vi "Word_Get_Table_Range.vi"(4 "end column":i32, 5 "start column":i32, 6 "end row":i32, 7 "start row":i32, 8 "error in":errorcluster, 9 "borders and shading":T1={"outside line style"=1, "outside color"=4278190080, "outside line width"=2, "inside line style"=1, "inside color"=4278190080, "inside line width"=2, "background pattern color"=4278190080} {"inside line style" items=["wdLineStyleNone", "wdLineStyleSingle", "wdLineStyleDot", "wdLineStyleDashSmallGap", "wdLineStyleDashLargeGap", "wdLineStyleDashDot", "wdLineStyleDashDotDot", "wdLineStyleDouble", "wdLineStyleTriple", "wdLineStyleThinThickSmallGap", "wdLineStyleThickThinSmallGap", "wdLineStyleThinThickThinSmallGap", "wdLineStyleThinThickMedGap", "wdLineStyleThickThinMedGap", "wdLineStyleThinThickThinMedGap", "wdLineStyleThinThickLargeGap", "wdLineStyleThickThinLargeGap", "wdLineStyleThinThickThinLargeGap", "wdLineStyleSingleWavy", "wdLineStyleDoubleWavy", "wdLineStyleDashDotStroked", "wdLineStyleEmboss3D", "wdLineStyleEngrave3D", "wdLineStyleOutset", "wdLineStyleInset"]; "inside line width" items=["wdLineWidth025pt"=2, "wdLineWidth050pt"=4, "wdLineWidth075pt"=6, "wdLineWidth100pt"=8, "wdLineWidth150pt"=12, "wdLineWidth225pt"=18, "wdLineWidth300pt"=24, "wdLineWidth450pt"=36, "wdLineWidth600pt"=48]; "outside line width" items=["wdLineWidth025pt"=2, "wdLineWidth050pt"=4, "wdLineWidth075pt"=6, "wdLineWidth100pt"=8, "wdLineWidth150pt"=12, "wdLineWidth225pt"=18, "wdLineWidth300pt"=24, "wdLineWidth450pt"=36, "wdLineWidth600pt"=48]; "outside line style" items=["wdLineStyleNone", "wdLineStyleSingle", "wdLineStyleDot", "wdLineStyleDashSmallGap", "wdLineStyleDashLargeGap", "wdLineStyleDashDot", "wdLineStyleDashDotDot", "wdLineStyleDouble", "wdLineStyleTriple", "wdLineStyleThinThickSmallGap", "wdLineStyleThickThinSmallGap", "wdLineStyleThinThickThinSmallGap", "wdLineStyleThinThickMedGap", "wdLineStyleThickThinMedGap", "wdLineStyleThinThickThinMedGap", "wdLineStyleThinThickLargeGap", "wdLineStyleThickThinLargeGap", "wdLineStyleThinThickThinLargeGap", "wdLineStyleSingleWavy", "wdLineStyleDoubleWavy", "wdLineStyleDashDotStroked", "wdLineStyleEmboss3D", "wdLineStyleEngrave3D", "wdLineStyleOutset", "wdLineStyleInset"]}, 10 "table":refnum<k7>, 11 "Word._Application":refnum<k7>) -> (0 "error out":errorcluster)   [LabVIEW 2010, in "NI_ReportGenerationToolkit.lvlib"]
uses:
  <vilib>/addons/_office/NI_ReportGenerationToolkit.lvlib
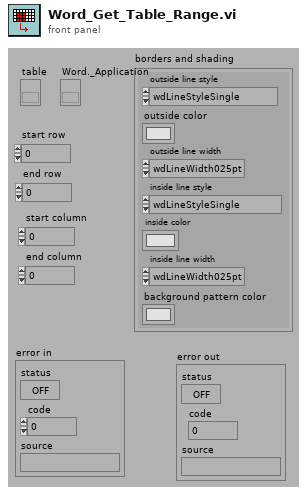
[diagram p1: front panel]
types:
  T1 = cluster{"outside line style":i32, "outside color":u32, "outside line width":i32, "inside line style":i32, "inside color":u32, "inside line width":i32, "background pattern color":u32}
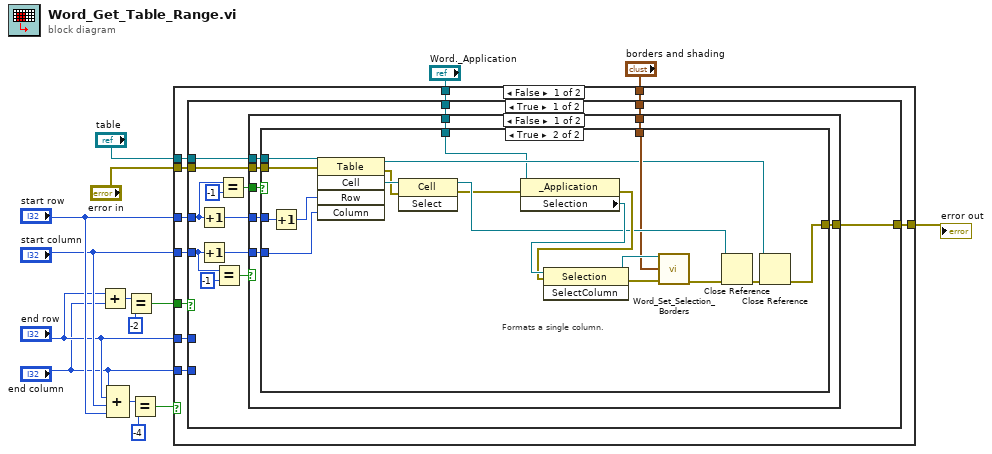
[diagram p0: block diagram]
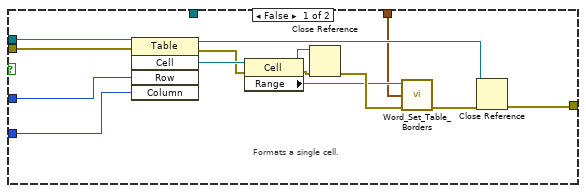
[diagram p2: hidden frame]
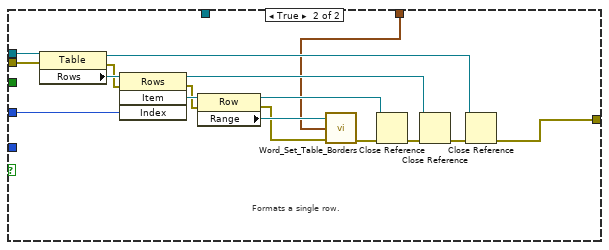
[diagram p3: hidden frame]
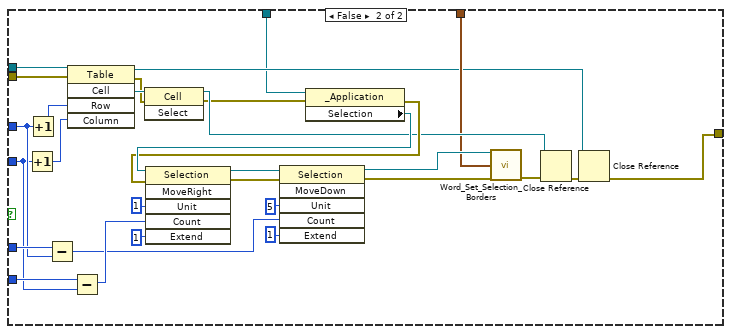
[diagram p4: hidden frame]
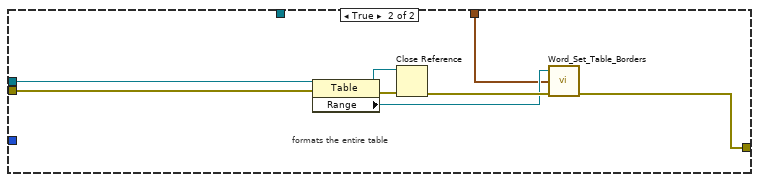
[diagram p5: hidden frame]
diagram:
  n1 = Add(x="end row", y="end column") -> (x+y=w13:i32)
  n2 = Compound Arithmetic op=ADD("end column", "end row", "start column", "start row") -> (w15:i32)
  n3 = Equal?(x=w13, y=-2) -> (x = y?=w4:bool)
  n4 = Equal?(x=w15, y=-4) -> (x = y?=w3:bool)
  n5 = case shown="False" w3 {
    tunnel: "start column" -> [w25 _]
    tunnel: "start row" -> [w24 _]
    tunnel: "end row" -> [w23 _]
    tunnel: "end column" -> [w22 _]
    tunnel: [w21 w128] -> w5
    tunnel: "table" -> [w20 w134]
    tunnel: "error in" -> [w19 w133]
    tunnel: "borders and shading" -> [w18 w127]
    tunnel: w4 -> [w17 _]
    tunnel: "Word._Application" -> [w16 _]
    frame False {
      n6 = case shown="True" w17 {
        tunnel: w25 -> [w32 w109]
        tunnel: w24 -> [w29 w110]
        tunnel: w23 -> [_ w112]
        tunnel: w22 -> [_ w111]
        tunnel: [w38 w104] -> w21
        tunnel: w20 -> [w37 w126]
        tunnel: w19 -> [w34 w125]
        tunnel: w18 -> [w27 w100]
        tunnel: w16 -> [w26 w97]
        frame True {
          n7 = Increment(x=w29) -> (x+1=w36:i32)
          n8 = Increment(x=w32) -> (x+1=w35:i32)
          n9 = Equal?(x=w32, y=-1) -> (x = y?=w33:bool)
          n10 = Equal?(x=w29, y=-1) -> (x = y?=w28:bool)
          n11 = case shown="False" w33 {
            tunnel: [w46 w85] -> w38
            tunnel: w37 -> [w45 w96]
            tunnel: w36 -> [w44 w94]
            tunnel: w35 -> [w43 _]
            tunnel: w34 -> [w42 w90]
            tunnel: w28 -> [w41 _]
            tunnel: w27 -> [w40 w80]
            tunnel: w26 -> [w39 _]
            frame False {
              n12 = case shown="True" w41 {
                tunnel: [w52 w72] -> w46
                tunnel: w45 -> [w58 w79]
                tunnel: w44 -> [w57 w77]
                tunnel: w43 -> [w56 w76]
                tunnel: w42 -> [w54 w78]
                tunnel: w40 -> [w47 w65]
                tunnel: w39 -> [_ w62]
                frame False {
                  # "Formats a single cell."
                  n13 = invoke class="Table" method="Cell"(reference=w58, error in=w54, "Row"=w57, "Column"=w56) -> (reference out=w51:refnum<k7>, error out=w53:errorcluster, "Cell"=w55:refnum<k7>)  [unwired: 1 in, 2 out]
                  n14 = property class="Cell"(reference=w55, error in=w53) -> (reference out=w60:refnum<k7>, error out=w59:errorcluster, "Range"=w48:refnum<k7>)
                  n15 = Close Reference(reference=w60, error in (no error)=w59) -> (error out=w49:errorcluster)
                  n16 = call <vilib>:"Word_Set_Table_Borders.vi"("range"=w48, "borders and shading"=w47, "error in"=w49) -> ("error out"=w50:errorcluster)  [unwired: 12 out]
                  n17 = Close Reference(reference=w51, error in (no error)=w50) -> (error out=w52:errorcluster)
                }
                frame True {
                  # "Formats a single column."
                  n18 = Increment(x=w77) -> (x+1=w61:i32)
                  n19 = invoke class="Table" method="Cell"(reference=w79, error in=w78, "Row"=w61, "Column"=w76) -> (reference out=w64:refnum<k7>, error out=w74:errorcluster, "Cell"=w75:refnum<k7>)  [unwired: 1 in, 2 out]
                  n20 = invoke class="Cell" method="Select"(reference=w75, error in=w74) -> (reference out=w69:refnum<k7>, error out=w63:errorcluster)  [unwired: 1 in, 1 out]
                  n21 = property class="_Application"(reference=w62, error in=w63) -> (error out=w70:errorcluster, "Selection"=w71:refnum<k7>)  [unwired: 1 out]
                  n22 = invoke class="Selection" method="SelectColumn"(reference=w71, error in=w70) -> (reference out=w66:refnum<k7>, error out=w68:errorcluster)  [unwired: 1 in, 1 out]
                  n23 = call <vilib>:"Word_Set_Selection_Borders.vi"("Word.Selection"=w66, "borders and shading"=w65, "error in"=w68) -> ("error out"=w67:errorcluster)  [unwired: 12 out]
                  n24 = Close Reference(reference=w69, error in (no error)=w67) -> (error out=w73:errorcluster)
                  n25 = Close Reference(reference=w64, error in (no error)=w73) -> (error out=w72:errorcluster)
                }
              }
            }
            frame True {
              # "Formats a single row."
              n26 = property class="Table"(reference=w96, error in=w90) -> (reference out=w84:refnum<k7>, error out=w92:errorcluster, "Rows"=w95:refnum<k7>)
              n27 = invoke class="Rows" method="Item"(reference=w95, error in=w92, "Index"=w94) -> (reference out=w87:refnum<k7>, error out=w91:errorcluster, "Item"=w93:refnum<k7>)  [unwired: 1 in, 1 out]
              n28 = property class="Row"(reference=w93, error in=w91) -> (reference out=w88:refnum<k7>, error out=w81:errorcluster, "Range"=w82:refnum<k7>)
              n29 = call <vilib>:"Word_Set_Table_Borders.vi"("range"=w82, "borders and shading"=w80, "error in"=w81) -> ("error out"=w83:errorcluster)  [unwired: 12 out]
              n30 = Close Reference(reference=w88, error in (no error)=w83) -> (error out=w89:errorcluster)
              n31 = Close Reference(reference=w87, error in (no error)=w89) -> (error out=w86:errorcluster)
              n32 = Close Reference(reference=w84, error in (no error)=w86) -> (error out=w85:errorcluster)
            }
          }
        }
        frame False {
          n33 = Increment(x=w109) -> (x+1=w123:i32)
          n34 = Increment(x=w110) -> (x+1=w124:i32)
          n35 = Subtract(x=w112, y=w110) -> (x-y=w107:i32)
          n36 = invoke class="Table" method="Cell"(reference=w126, error in=w125, "Row"=w124, "Column"=w123) -> (reference out=w98:refnum<k7>, error out=w121:errorcluster, "Cell"=w122:refnum<k7>)  [unwired: 1 in, 2 out]
          n37 = Subtract(x=w111, y=w109) -> (x-y=w108:i32)
          n38 = invoke class="Cell" method="Select"(reference=w122, error in=w121) -> (reference out=w105:refnum<k7>, error out=w99:errorcluster)  [unwired: 1 in, 1 out]
          n39 = property class="_Application"(reference=w97, error in=w99) -> (error out=w119:errorcluster, "Selection"=w120:refnum<k7>)  [unwired: 1 out]
          n40 = invoke class="Selection" method="MoveRight"(reference=w120, error in=w119, "Unit"=1, "Count"=w108, "Extend"=1) -> (reference out=w116:refnum<k7>, error out=w115:errorcluster)  [unwired: 1 in, 4 out]
          n41 = invoke class="Selection" method="MoveDown"(reference=w116, error in=w115, "Unit"=5, "Count"=w107, "Extend"=1) -> (reference out=w101:refnum<k7>, error out=w102:errorcluster)  [unwired: 1 in, 4 out]
          n42 = call <vilib>:"Word_Set_Selection_Borders.vi"("Word.Selection"=w101, "borders and shading"=w100, "error in"=w102) -> ("error out"=w103:errorcluster)  [unwired: 12 out]
          n43 = Close Reference(reference=w105, error in (no error)=w103) -> (error out=w106:errorcluster)
          n44 = Close Reference(reference=w98, error in (no error)=w106) -> (error out=w104:errorcluster)
        }
      }
    }
    frame True {
      # "formats the entire table"
      n45 = property class="Table"(reference=w134, error in=w133) -> (reference out=w131:refnum<k7>, error out=w132:errorcluster, "Range"=w129:refnum<k7>)
      n46 = Close Reference(reference=w131, error in (no error)=w132) -> (error out=w130:errorcluster)
      n47 = call <vilib>:"Word_Set_Table_Borders.vi"("range"=w129, "borders and shading"=w127, "error in"=w130) -> ("error out"=w128:errorcluster)  [unwired: 12 out]
    }
  }
  "error out" <- w5
